vi "Get File Feature.vi"(8 "error in (no error)":errorcluster, 11 "String":string) -> (0 "error out":errorcluster, 1 "File type":string, 2 "Filename":string, 3 "Folder":string)   [LabVIEW 2017, in "File.lvlib"]
uses:
  File.lvlib
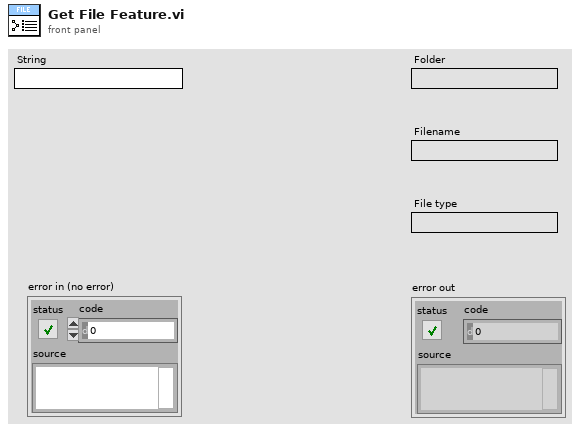
[diagram p1: front panel]
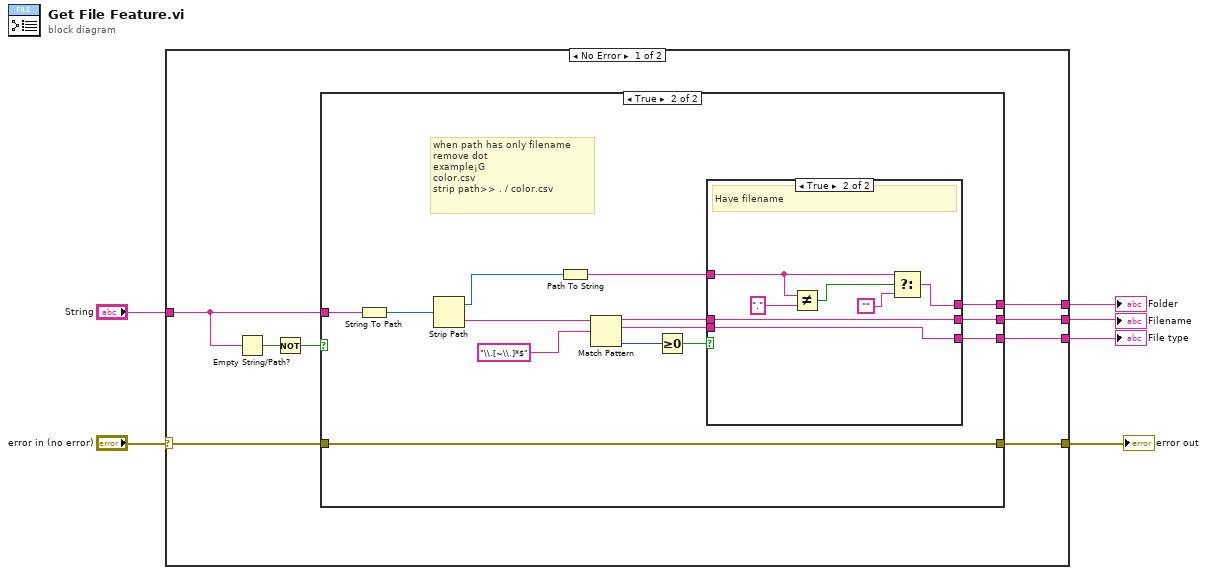
[diagram p0: block diagram]
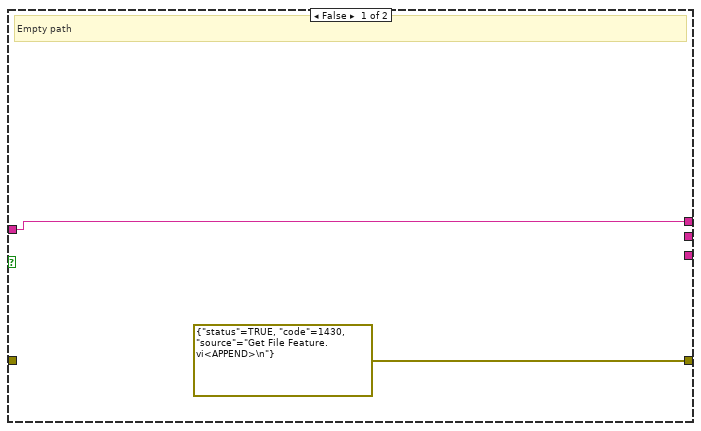
[diagram p2: hidden frame]
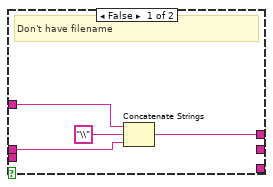
[diagram p3: hidden frame]
diagram:
  n1 = case shown="No Error" "error in (no error)" {
    selector: "error in (no error)" -> [w9 w42]
    tunnel: "String" -> [w14 w43]
    tunnel: [w11 w43] -> w6
    tunnel: [w10 w42] -> w4
    tunnel: [w8 _] -> w2
    tunnel: [w7 _] -> w1
    frame No Error {
      n2 = Empty String/Path?(string/path=w14) -> (empty?=w13:bool)
      n3 = Not(x=w13) -> (.not. x?=w12:bool)
      n4 = case shown="True" w12 {
        tunnel: w14 -> [w16 w30]
        tunnel: [w16 w19] -> w11
        tunnel: [errorcluster {"status"=TRUE, "code"=1430, "source"="Get File Feature.vi<APPEND>\n"} ("error out 2") w26] -> w10
        tunnel: w9 -> [_ w26]
        tunnel: [_ w18] -> w8
        tunnel: [_ w17] -> w7
        frame False {
          # "Empty path"
        }
        frame True {
          # "when path has only filename\nremove dot\nexample¡G\ncolor.csv\nstrip path>> . / color.csv"
          n5 = String To Path(string=w30) -> (path=w27:path)
          n6 = Strip Path(path=w27) -> (stripped path=w24:path, name=w29:string)
          n7 = Path To String(path=w24) -> (string=w22:string)
          n8 = Match Pattern(string=w29, regular expression="\\.[~\\.]*$") -> (before substring=w21:string, match substring=w20:string, offset past match=w25:i32)  [unwired: 1 in, 1 out]
          n9 = Greater Or Equal To 0?(x=w25) -> (x >= 0?=w23:bool)
          n10 = case shown="True" w23 {
            tunnel: w22 -> [w33 w37]
            tunnel: w21 -> [w34 w41]
            tunnel: w20 -> [_ w40]
            tunnel: [w32 w36] -> w19
            tunnel: [_ w41] -> w18
            tunnel: [_ w40] -> w17
            frame False {
              # "Don't have filename"
              n11 = Concatenate Strings(w33, "\\", w34) -> (w32:string)
            }
            frame True {
              # "Have filename"
              n12 = Not Equal?(x=w37, y=".") -> (x != y?=w38:bool)
              n13 = Select(t=w37, s=w38, f="") -> (s? t:f=w36:string)
            }
          }
        }
      }
    }
    frame Error {
    }
  }
  "Filename" <- w2
  "File type" <- w1
  "Folder" <- w6
  "error out" <- w4
